vi "PH_SSAC.c in mm per fs.vi"() -> (0 "c [mm/fs]":dbl)   [LabVIEW 2014, in "PH_SSAC.lvlib"]
doc: "This is the speed of light in mm/fs."
uses:
  PH_SSAC.lvlib
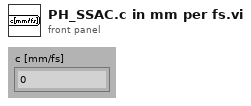
[diagram p1: front panel]
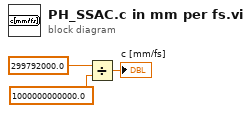
[diagram p0: block diagram]
diagram:
  n1 = Divide(x=299792000.0, y=1000000000000.0) -> (x/y=→"c [mm/fs]":dbl)
